vi "Status RefrigOpState.vi"(8 "error in (no error)":errorcluster, 10 "Address (0)":i32, 11 "VISA resource name":refnum<visa-resource-name>) -> (0 "error out":errorcluster, 1 "Operation state":bool[](array[boolean]), 2 "#Refrigerators":u8, 3 "VISA resource name out":refnum<visa-resource-name>)   [LabVIEW 2016, in "Environment Chamber.lvlib" / "Climatic Chamber.lvlib"]
doc: "<b>Refrigeration output monitor</B>\n\nReturns the number of equipped refrigerators and their operation state."
uses:
  Climatic Chamber.lvlib
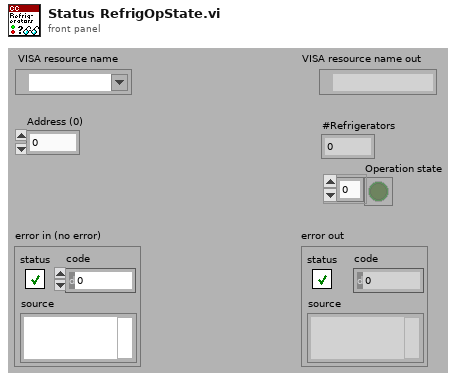
[diagram p1: front panel]
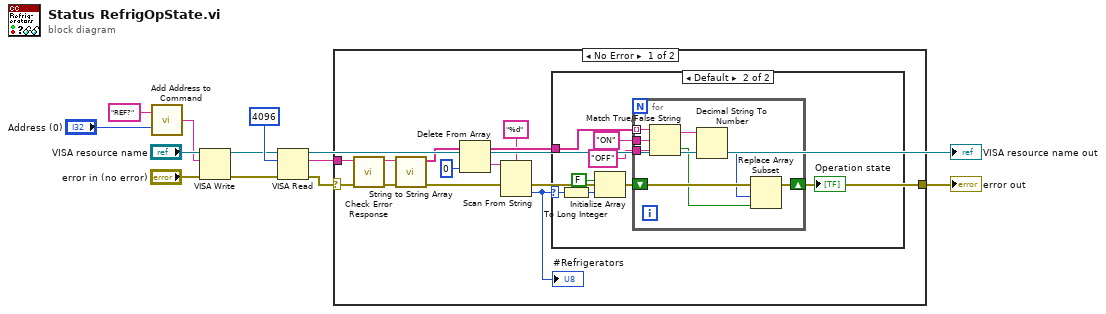
[diagram p0: block diagram]
diagram:
  n1 = call "Add Address to Command.vi"("Address (0)"="Address (0)", "Command"="REF?") -> ("Command OUT"=w5:string)
  n2 = VISA Write(VISA resource name="VISA resource name", write buffer=w5, error in (no error)="error in (no error)") -> (VISA resource name out=w9:refnum<visa-resource-name>, error out=w8:errorcluster)  [unwired: 1 out]
  n3 = VISA Read(VISA resource name=w9, byte count=u32 4096, error in (no error)=w8) -> (VISA resource name out=→"VISA resource name out":refnum<visa-resource-name>, read buffer=w3:string, error out=w4:errorcluster)  [unwired: 1 out]
  n4 = case shown="No Error" w4 {
    selector: w4 -> [w22 w41]
    tunnel: w3 -> [w23 _]
    tunnel: [w19 w41] -> w2
    frame No Error {
      n5 = call "Check Error Response.vi"("error in (no error)"=w22, "read String"=w23) -> ("error out"=w20:errorcluster, "String out"=w17:string)  [unwired: 7 in, 1 out]
      n6 = call "String to String Array.vi"("error in (no error)"=w20, "String received"=w17) -> ("error out"=w18:errorcluster, "Array Data"=w16:string[])  [unwired: 8 in]
      n7 = Delete From Array(array=w16, index=0) -> (deleted portion=w15:string, array with subset deleted=w24:string[])  [unwired: 1 in]
      n8 = Scan From String(format string="%d", input string=w15, error in=w18) -> (error out=w19:errorcluster, output 1=w13:u8)  [unwired: 2 in, 2 out]
      "#Refrigerators" <- w13
      n9 = case shown="Default" w13 {
        selector: w13 -> [_ w32]
        tunnel: w24 -> [_ w28]
        frame 0 {
        }
        frame Default {
          n10 = To Long Integer(number=w32) -> (32bit integer=w31:i32)
          n11 = Initialize Array(FALSE, w31) -> (w29:bool[])
          n12 = for {
            shift-right: [w36] -> w25
            shift-left: w29 -> [w37]
            tunnel: w28 -> [w40] mode=indexing
            tunnel: "ON" ("true string") -> [w39]
            tunnel: "OFF" ("true string") -> [w38]
            n13 = Match True/False String(2:w38, 3:w39, 4:w40) -> (0:w33:bool, 1:w35:string)
            n14 = Decimal String To Number(string=w35) -> (number=w34:i32)  [unwired: 2 in, 1 out]
            n15 = Replace Array Subset(array=w37, new element=w33, index=w34) -> (w36:bool[])
          }
          "Operation state" <- w25
        }
      }
    }
    frame Error {
    }
  }
  "error out" <- w2
